vi "PID-Analog PWM-Encoder.vi"() -> ()   [LabVIEW 2021]
uses:
  <vilib>/DAQmx/read.llb/DAQmx Read (Counter DBL 1Chan 1Samp).vi
  <vilib>/DAQmx/write.llb/DAQmx Write (Analog 1D DBL 1Chan NSamp).vi
  <vilib>/DAQmx/create/channels.llb/DAQmx Create Channel (AO-Voltage-Basic).vi
  <vilib>/DAQmx/create/channels.llb/DAQmx Create Channel (CI-Position-Angular Encoder).vi
  <vilib>/DAQmx/miscellaneous.llb/DAQmx Fill In Error Info.vi
  <vilib>/addons/control/pid/pid.llb/PID (DBL).vi
  <vilib>/measure/NI_MABase.lvlib
  <vilib>/addons/control/pid/NI_PID_pid.lvlib
  <resource>/objmgr/daqmx.rc
panel:
  in  "Pulses Per Revolution":u32=24
  in  "B Input Terminal":tag="PFI10"
  in  "A Input Terminal":tag="PFI8"
  in  "Counter":tag="Dev1/ctr0"
  in  "PID Gains":T1={"proportional gain (Kc)"=1.0, "integral time (Ti, min)"=0.01, "derivative time (Td, min)"=0.0} {"derivative time (Td, min)" format="%.3f"; "integral time (Ti, min)" format="%.3f"; "proportional gain (Kc)" format="%.3f"}
  in  "Rotation target\n(deg)":dbl
  in  "PWM Control (Analog Out)":tag="myDAQ1/ao1"
  in  "?":bool
  out "PWM Control Signal":waveform(dbl)(graph)={"t0"=timestamp(0 s since 1904-01-01), "dt"=0.001, "Y"=[0.0, 0.0, 0.0, 0.0, 0.0, 0.0, 0.0, 0.0, 0.0, 0.0, 0.0, 0.0, 0.0, 0.0, 0.0, 0.0, 0.0, 0.0, 0.0, 0.0, 0.0, 0.0, 0.0, 0.0, 0.0, 0.0, 0.0, 0.0, 0.0, 0.0, 0.0, 0.0, 0.0, 0.0, 0.0, 0.0, 0.0, 0.0, 0.0, 0.0, 0.0, 0.0, 0.0, 0.0, 0.0, 0.0, 0.0, 0.0, 0.0, 0.0]}
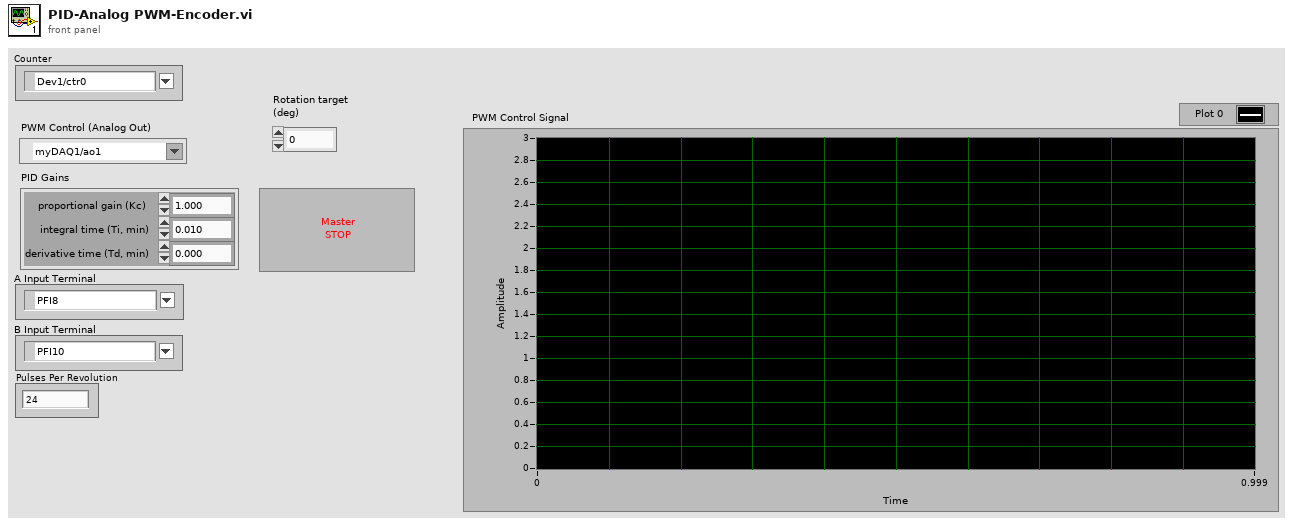
[diagram p1: front panel]
types:
  T1 = cluster{"proportional gain (Kc)":dbl, "integral time (Ti, min)":dbl, "derivative time (Td, min)":dbl}
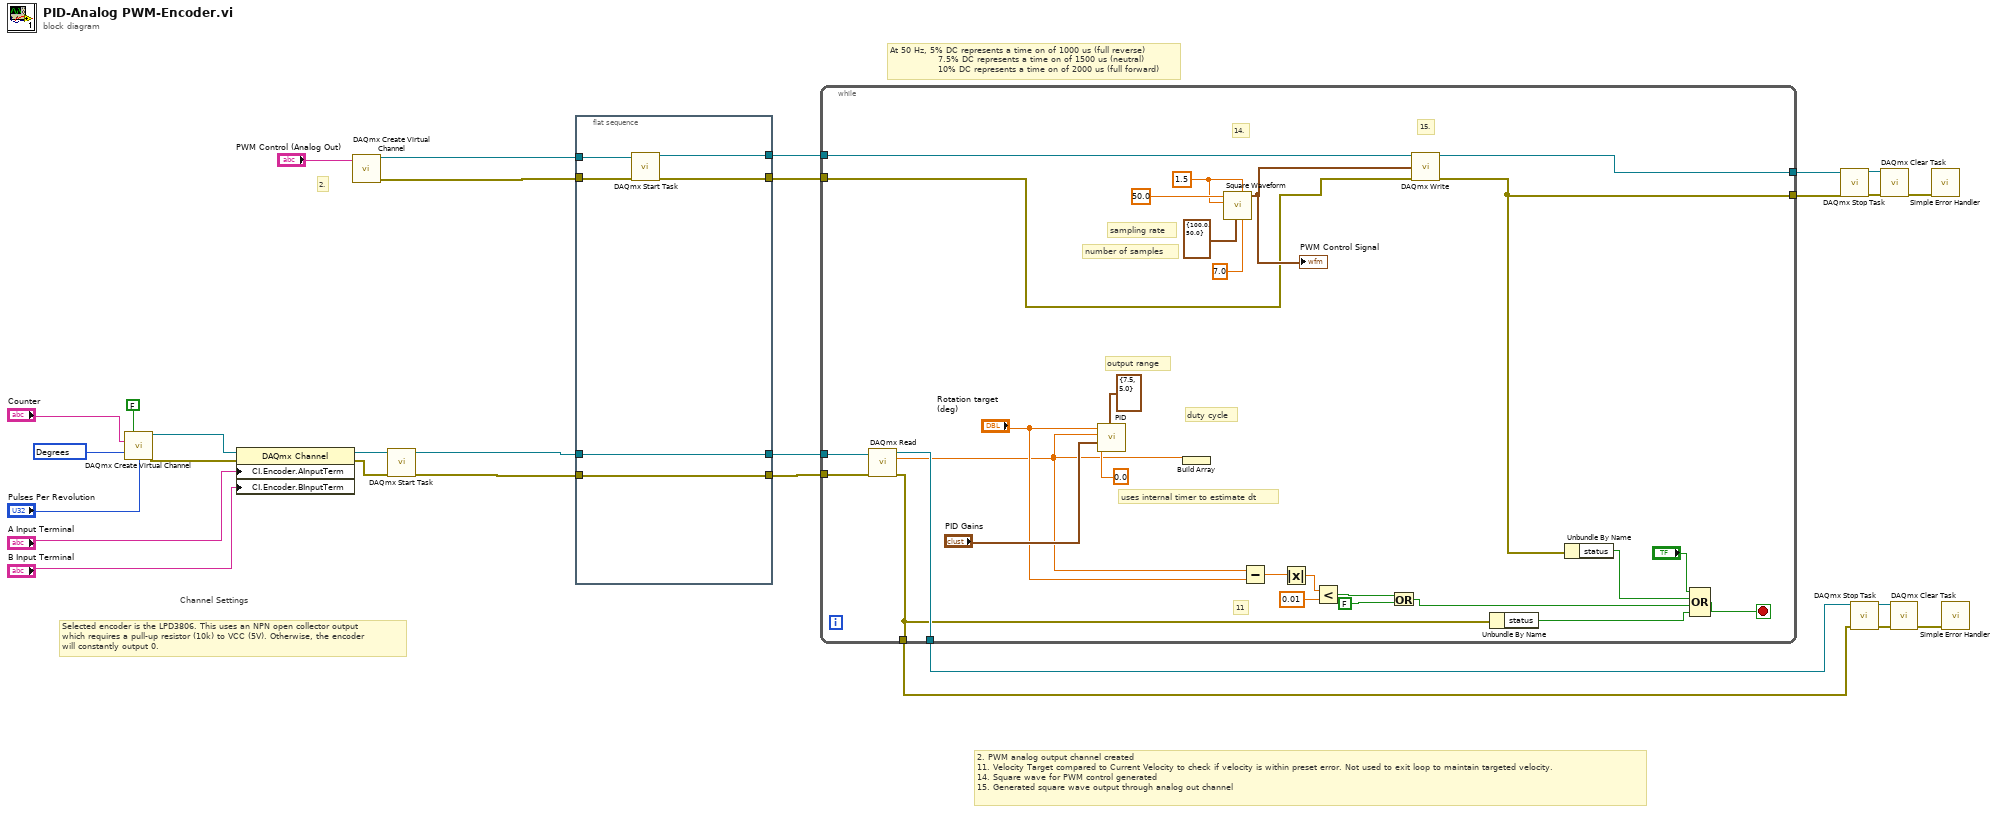
[diagram p0: block diagram]
diagram:
  w2 = 10146 items=["Degrees"=10146, "Radians"=10273, "Ticks"=10304, "From Custom Scale"=10065] ("units")
  # "At 50 Hz, 5% DC represents a time on of 1000 us (full reverse)\n                7.5% DC represents a time on of 1500 us (neutral)\n                10% DC represents a time on of 2000 us (full forward)"
  # "Channel Settings"
  # "Selected encoder is the LPD3806. This uses an NPN open collector output\nwhich requires a pull-up resistor (10k) to VCC (5V). Otherwise, the encoder\nwill constantly output 0."
  # "2. PWM analog output channel created\n11. Velocity Target compared to Current Velocity to check if velocity is within preset error. Not used to exit loop to maintain targeted velocity.\n14. Square wave for PWM control generated\n15. Generated square wave output through analog out channel"
  # "2."
  n1 = call-poly <vilib>:"DAQmx Create Virtual Channel.vi"("z index enable"=FALSE, "counter"="Counter", "units"=w2, "pulses per revolution"="Pulses Per Revolution") -> ("task out"=w18:refnum<k21>, "error out"=w17:errorcluster)  [unwired: 10 in]
  n2 = property class="DAQmx Channel"(reference=w18, error in=w17, "CI.Encoder.AInputTerm"="A Input Terminal", "CI.Encoder.BInputTerm"="B Input Terminal") -> (reference out=w13:refnum<k21>, error out=w12:errorcluster)
  n3 = call-poly <vilib>:"DAQmx Create Virtual Channel.vi"("physical channels"="PWM Control (Analog Out)") -> ("task out"=w25:refnum<k21>, "error out"=w24:errorcluster)  [unwired: 13 in]
  n4 = call <vilib>:"DAQmx Start Task.vi"("task/channels in"=w13, "error in"=w12) -> ("task out"=w10:refnum<k21>, "error out"=w8:errorcluster)  [unwired: 12 in]
  n5 = flat-sequence {
    tunnel: [w35] -> w29
    tunnel: w25 -> [w34]
    tunnel: w24 -> [w33]
    tunnel: [w32] -> w23
    tunnel: [w31] -> w11
    tunnel: w10 -> [w31]
    tunnel: [w30] -> w9
    tunnel: w8 -> [w30]
    frame #0 {
      n6 = call <vilib>:"DAQmx Start Task.vi"("task/channels in"=w34, "error in"=w33) -> ("task out"=w35:refnum<k21>, "error out"=w32:errorcluster)  [unwired: 12 in]
    }
  }
  n7 = while {
    tunnel: w29 -> [w63]
    tunnel: [w62] -> w21
    tunnel: [w56] -> w20
    tunnel: w23 -> [w50]
    tunnel: w9 -> [w48]
    tunnel: w11 -> [w47]
    tunnel: [w41] -> w4
    tunnel: [w46] -> w3
    stop <- w45 stop-if-true
    w58 = 1.5 ("amplitude")
    # "duty cycle"
    # "uses internal timer to estimate dt"
    # "output range"
    # "number of samples"
    # "sampling rate"
    # "11"
    # "15."
    # "14."
    n8 = call-poly <vilib>:"DAQmx Read.vi"("task/channels in"=w47, "error in"=w48) -> ("task out"=w46:refnum<k21>, "data"=w37:dbl, "error out"=w41:errorcluster)  [unwired: 11 in]
    n9 = call-poly <vilib>:"PID.vi"("output range"=cluster{"output high":dbl, "output low":dbl} {"output high"=7.5, "output low"=5.0}, "dt (s)"=0.0, "PID gains"="PID Gains", "process variable"=w37, "setpoint"="Rotation target\n(deg)") -> ()  [unwired: 5 in, 2 out]
    n10 = Build Array(w37) -> ()  [unwired: 1 out]
    n11 = call <vilib>:"Square Waveform.vi"("duty cycle (%)"=7.0, "offset"=w58, "sampling info"=cluster{"Fs":dbl, "#s":dbl} {"Fs"=100.0, "#s"=50.0}, "amplitude"=w58, "frequency"=50.0) -> ("signal out"=w61:waveform(dbl))  [unwired: 5 in, 1 out]
    "PWM Control Signal" <- w61
    n12 = Subtract(x=w37, y="Rotation target\n(deg)") -> (x-y=w53:dbl)
    n13 = Absolute Value(x=w53) -> (abs(x)=w52:dbl)
    n14 = Less?(x=w52, y=0.01) -> (x < y?=w39:bool)
    n15 = Or(x=w39, y=FALSE) -> (x .or. y?=w38:bool)
    n16 = call-poly <vilib>:"DAQmx Write.vi"("task/channels in"=w63, "data"=w61, "error in"=w50) -> ("task out"=w62:refnum<k21>, "error out"=w56:errorcluster)  [unwired: 10 in, 1 out]
    n17 = Unbundle By Name(w41) -> ("status"=w42:bool)
    n18 = Unbundle By Name(w56) -> ("status"=w43:bool)
    n19 = Compound Arithmetic op=OR("?", w43, w38, w42) -> (w45:bool)
  }
  n20 = call <vilib>:"DAQmx Stop Task.vi"("task/channels in"=w21, "error in"=w20) -> ("task out"=w28:refnum<k21>, "error out"=w27:errorcluster)  [unwired: 12 in]
  n21 = call <vilib>:"DAQmx Stop Task.vi"("task/channels in"=w3, "error in"=w4) -> ("task out"=w7:refnum<k21>, "error out"=w6:errorcluster)  [unwired: 12 in]
  n22 = call <vilib>:"DAQmx Clear Task.vi"("task in"=w28, "error in"=w27) -> ("error out"=w22:errorcluster)  [unwired: 13 in]
  n23 = call <vilib>:"DAQmx Clear Task.vi"("task in"=w7, "error in"=w6) -> ("error out"=w5:errorcluster)  [unwired: 13 in]
  n24 = call <vilib>:"Simple Error Handler.vi"("error in (no error)"=w22) -> ()  [unwired: 4 in, 5 out]
  n25 = call <vilib>:"Simple Error Handler.vi"("error in (no error)"=w5) -> ()  [unwired: 4 in, 5 out]
